vi "Sheet String To Array.vi"(10 "Sheet String":string) -> (2 "Table Array":string[](array[string]))   [LabVIEW 2018, in "Agilent U2000 Series.lvlib"]
doc: "Parses the sheet format string returned by instrument to an array of string."
uses:
  Agilent U2000 Series.lvlib
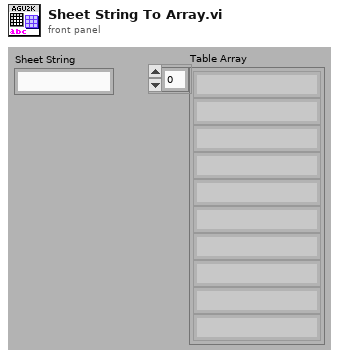
[diagram p1: front panel]
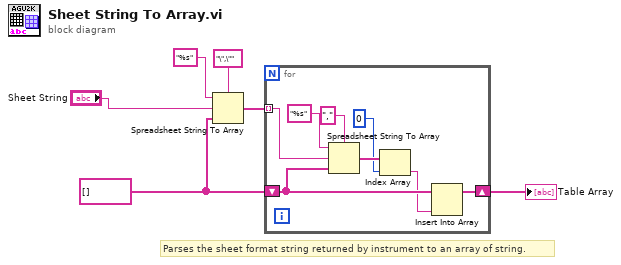
[diagram p0: block diagram]
diagram:
  w3 = string[] []
  # "Parses the sheet format string returned by instrument to an array of string."
  n1 = Spreadsheet String To Array(delimiter (Tab)="\",\"", format string="%s", spreadsheet string="Sheet String", array type (2D Dbl)=w3) -> (array=w4:string[])
  n2 = for {
    tunnel: w4 -> [w8] mode=indexing
    shift-right: [w14] -> w2
    shift-left: w3 -> [w12]
    n3 = Spreadsheet String To Array(delimiter (Tab)=",", format string="%s", spreadsheet string=w8, array type (2D Dbl)=w12) -> (array=w11:string[])
    n4 = Index Array(array=w11, index=0) -> (element=w9:string)
    n5 = Insert Into Array(array=w12, new element=w9) -> (w14:string[])  [unwired: 1 in]
  }
  "Table Array" <- w2
